vi "Add Header.vi"(8 "error in (no error)":errorcluster, 11 "Text File Sink in":refnum<class "Text File Sink.lvclass">) -> (0 "error out":errorcluster, 3 "Text File Sink out":refnum<class "Text File Sink.lvclass">)   [LabVIEW 2019, in "Text File Sink.lvclass"]
doc: "--\nCopyright © 2017 Composed SystemsI All rights reserved.\n\nAuthor: Jon McBee <jon.mcbee@composed.io>\n\nThis library is provided \"AS IS\" ,WITHOUT WARRANTIES OR\nCONDITIONS OF ANY KIND, either express or implied.\n\nComposed Systems -- composed.io\n\nStream 0.0.1.1\nJon McBee - Composed Systems\nCopyright (c) 2017, Composed Systems"
uses:
  <vilib>/gpm_packages/@cs/event-logger/Source/Text File Sink/Text File Sink.lvclass
  <vilib>/gpm_packages/@cs/event-logger/Source/Text File Sink/Text File Sink.lvclass/Text File Sink.ctl
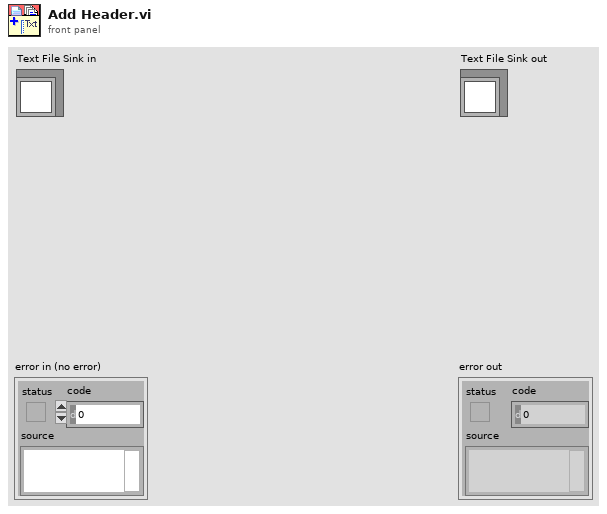
[diagram p1: front panel]
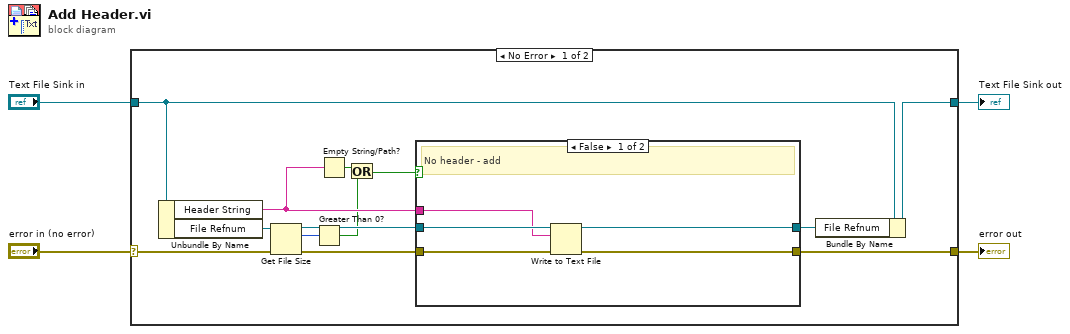
[diagram p0: block diagram]
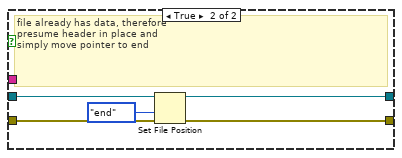
[diagram p2: hidden frame]
diagram:
  n1 = case shown="No Error" "error in (no error)" {
    selector: "error in (no error)" -> [w12 w29]
    tunnel: [w10 w29] -> w3
    tunnel: [w11 w28] -> w1
    tunnel: "Text File Sink in" -> [w9 w28]
    frame No Error {
      n2 = Unbundle By Name(w9) -> ("Header String"=w8:string, "File Refnum"=w14:refnum<file>)
      n3 = Get File Size(file=w14, error in=w12) -> (refnum out=w15:refnum<file>, size (in bytes)=w17:i64, 0:w16:errorcluster)
      n4 = Greater Than 0?(x=w17) -> (x > 0?=w6:bool)
      n5 = Empty String/Path?(string/path=w8) -> (empty?=w7:bool)
      n6 = Or(x=w7, y=w6) -> (x .or. y?=w5:bool)
      n7 = case shown="False" w5 {
        tunnel: w16 -> [w22 w27]
        tunnel: w15 -> [w21 w26]
        tunnel: [w19 w24] -> w10
        tunnel: [w20 w23] -> w13
        tunnel: w8 -> [w18 _]
        frame False {
          # "No header - add"
          n8 = Write to Text File(file (use dialog)=w21, text=w18, error in=w22) -> (refnum out=w20:refnum<file>, error out=w19:errorcluster)  [unwired: 2 out]
        }
        frame True {
          # "file already has data, therefore\npresume header in place and\nsimply move pointer to end"
          n9 = Set File Position(refnum=w26, from (0:start)=enum16{"start", "end", "current"}."end", error in=w27) -> (refnum out=w23:refnum<file>, error out=w24:errorcluster)  [unwired: 1 out]
        }
      }
      n10 = Bundle By Name(cluster=w9, "File Refnum"=w13) -> (w11:refnum<class "Text File Sink.lvclass">)
    }
    frame Error {
    }
  }
  "error out" <- w3
  "Text File Sink out" <- w1
